vi "Force Calibration Chart.vi"() -> ()   [LabVIEW 2020]
uses:
  Inflation Test/Result Handling/Inflation Test Numeric Results.ctl
panel:
  out "Current Force":cluster{dbl[], dbl[]}(graph)
  out "Calibration Equations":cluster{dbl[], dbl[]}[](graph)
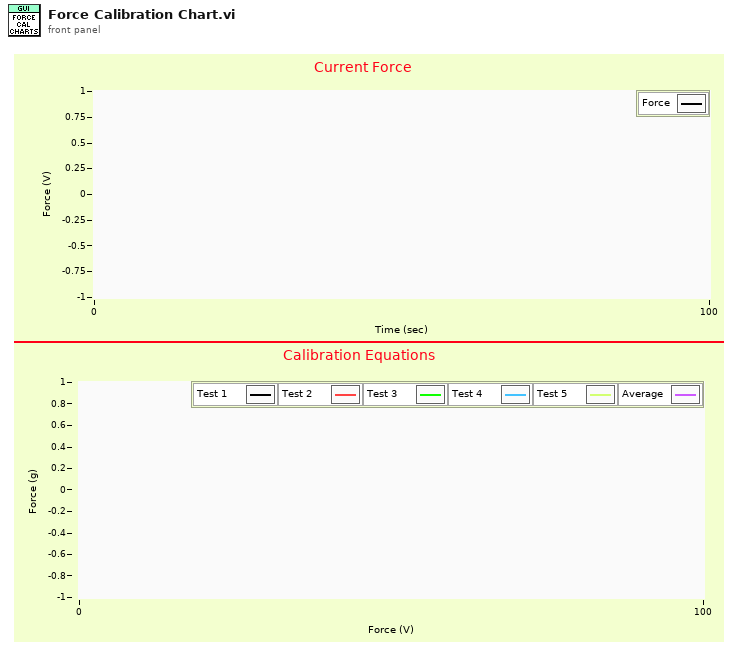
[diagram p1: front panel]
types:
  T1 = typedef "Inflation Test Numeric Results.ctl" = cluster{"diameter":dbl, "diameter time":dbl, "force":dbl, "force time":dbl, "setpoint":dbl}
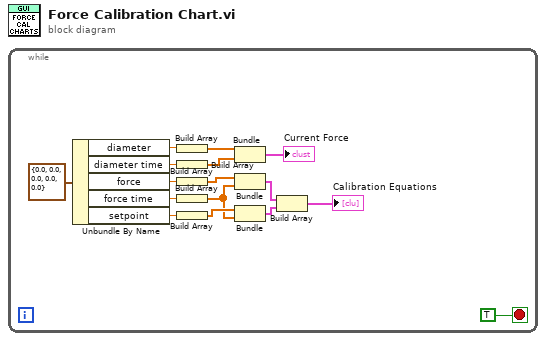
[diagram p0: block diagram]
diagram:
  n1 = while {
    stop <- TRUE stop-if-true
    n2 = Unbundle By Name(T1 {"diameter"=0.0, "diameter time"=0.0, "force"=0.0, "force time"=0.0, "setpoint"=0.0}) -> ("diameter"=w14:dbl, "diameter time"=w12:dbl, "force"=w10:dbl, "force time"=w11:dbl, "setpoint"=w13:dbl)
    n3 = Build Array(w14) -> (w9:dbl[])
    n4 = Build Array(w12) -> (w8:dbl[])
    n5 = Build Array(w10) -> (w6:dbl[])
    n6 = Build Array(w11) -> (w4:dbl[])
    n7 = Build Array(w13) -> (w5:dbl[])
    n8 = Bundle(w9, w8) -> (→"Current Force":cluster{dbl[], dbl[]})  [unwired: 1 in]
    n9 = Bundle(w6, w4) -> (w3:cluster{dbl[], dbl[]})  [unwired: 1 in]
    n10 = Bundle(w5, w4) -> (w2:cluster{dbl[], dbl[]})  [unwired: 1 in]
    n11 = Build Array(w3, w2) -> (→"Calibration Equations":cluster{dbl[], dbl[]}[])
  }
